vi "Furnace PID 20150313.vi"(4 "PID gains":T1={"proportional gain (Kc)"=1.0, "integral time (Ti, min)"=0.1, "derivative time (Td, min)"=0.0}, 5 "Furnace Baseline":dbl format="%.2f", 6 "PV Furnace degC":dbl format="%.2f", 7 "Counter Interval":i32, 8 "PV Bed degC":dbl format="%.2f", 9 "SP Bed DegC":dbl format="%.2f", 10 "Furnace SP":dbl format="%.2f", 11 "Counter In":i32) -> (2 "Furnace SP":dbl format="%.2f", 3 "Counter Out":i32)   [LabVIEW 2014]
uses:
  <vilib>/addons/control/pid/pid.llb/PID (DBL).vi
  <vilib>/addons/control/pid/NI_PID_pid.lvlib
panel:
  in  "output range":cluster{"output high":dbl, "output low":dbl}={"output high"=100.0, "output low"=-100.0} {"output low" format="%.2f"; "output high" format="%.2f"}
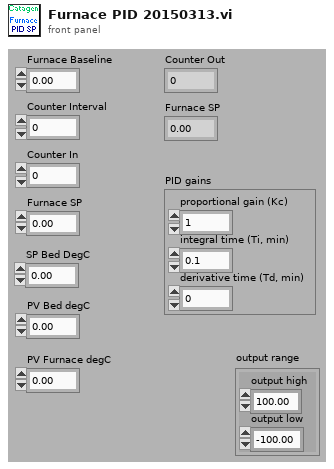
[diagram p1: front panel]
types:
  T1 = cluster{"proportional gain (Kc)":dbl, "integral time (Ti, min)":dbl, "derivative time (Td, min)":dbl}
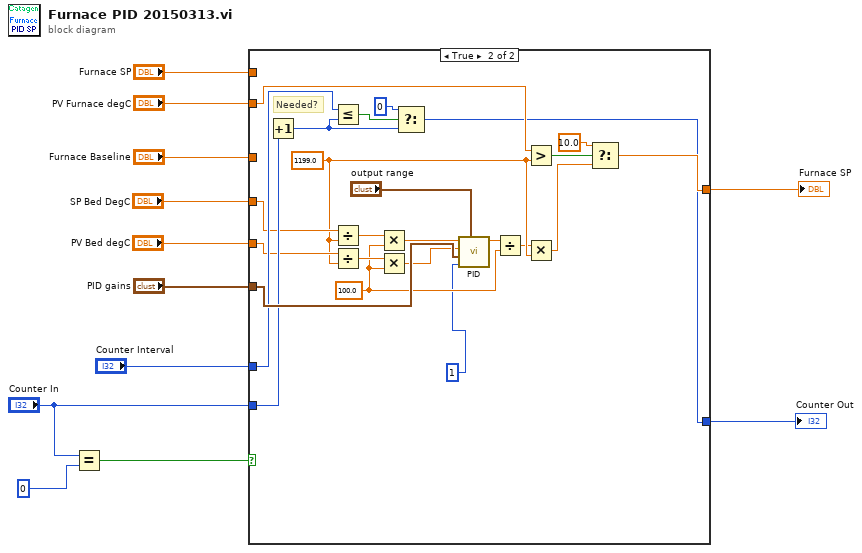
[diagram p0: block diagram]
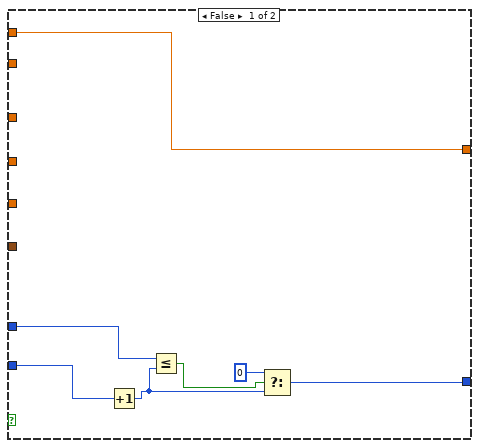
[diagram p2: hidden frame]
diagram:
  n1 = Equal?(x="Counter In", y=0) -> (x = y?=w2:bool)
  n2 = case shown="True" w2 {
    tunnel: "PID gains" -> [_ w43]
    tunnel: "PV Bed degC" -> [_ w32]
    tunnel: "PV Furnace degC" -> [_ w42]
    tunnel: [w19 w41] -> w9
    tunnel: "SP Bed DegC" -> [_ w33]
    tunnel: "Furnace Baseline" -> [_ _]
    tunnel: "Furnace SP" -> [w19 _]
    tunnel: "Counter Interval" -> [w15 w36]
    tunnel: "Counter In" -> [w14 w35]
    tunnel: [w13 w34] -> w1
    frame False {
      n3 = Increment(x=w14) -> (x+1=w17:i32)
      n4 = Less Or Equal?(x=w15, y=w17) -> (x <= y?=w16:bool)
      n5 = Select(t=0, s=w16, f=w17) -> (s? t:f=w13:i32)
    }
    frame True {
      w24 = 100.0 ("y")
      w23 = 1199.0 ("y")
      # "Needed?"
      n6 = Increment(x=w35) -> (x+1=w38:i32)
      n7 = Less Or Equal?(x=w36, y=w38) -> (x <= y?=w37:bool)
      n8 = Divide(x=w33, y=w23) -> (x/y=w31:dbl)
      n9 = Divide(x=w32, y=w23) -> (x/y=w30:dbl)
      n10 = Multiply(x=w31, y=w24) -> (x*y=w29:dbl)
      n11 = Multiply(x=w30, y=w24) -> (x*y=w28:dbl)
      n12 = Select(t=0, s=w37, f=w38) -> (s? t:f=w34:i32)
      n13 = call-poly <vilib>:"PID.vi"("output range"="output range", "dt (s)"=1 ("y"), "PID gains"=w43, "process variable"=w28, "setpoint"=w29) -> ("output"=w25:dbl)  [unwired: 5 in, 1 out]
      n14 = Divide(x=w25, y=w24) -> (x/y=w22:dbl)
      n15 = Greater?(x=w42, y=w23) -> (0:w40:bool)
      n16 = Multiply(x=w22, y=w23) -> (x*y=w21:dbl)
      n17 = Select(t=10.0, s=w40, f=w21) -> (s? t:f=w41:dbl)
    }
  }
  "Furnace SP" <- w9
  "Counter Out" <- w1
